vi "Register Events and Run.vi"(8 "error in (no error)":errorcluster, 11 "Panel in":refnum<class "Panel.lvclass">) -> (0 "error out":errorcluster, 2 "Panel Event Reg":refnum<event-registration>, 3 "Panel out":refnum<class "Panel.lvclass">)   [LabVIEW 2020, in "OOPanel.lvlib" / "Panel.lvclass"]
doc: "Simultaneously creates an event registration for the Panel events (Visibility, Close, etc) and marks the panel as running. Alternatively, Panel VIs can use the <b>Get Panel Events</b> property and then set the <b>Running</b> to true once the events are registered.\n\nFor more information on the <b>Running</b> property, see the VI documentation on <b>Set Running.vi</b>"
uses:
  Panel.lvclass
  Visibility State.ctl
  OOPanel.lvlib
  Visbility Event Data.ctl
  Panel Events.ctl
  Close Reason.ctl
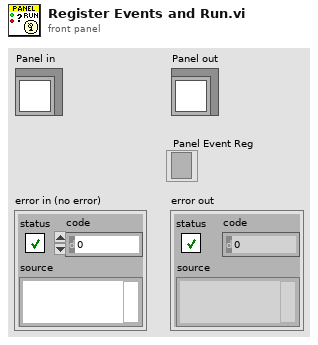
[diagram p1: front panel]
types:
  T1 = typedef "OOPanel.lvlib/Panel.lvclass/Panel Events.ctl" = cluster{"Visbility":refnum<user-event>, "Close":refnum<user-event>}
  T2 = typedef "OOPanel.lvlib/Panel.lvclass/Ref Data.ctl" = cluster{"Panel Ref":refnum<vi>, "SubPanel":refnum<vi>, "Close":bool, "Running":bool, "State":T3}
  T3 = typedef "OOPanel.lvlib/Visibility State.ctl" = enum16{"Idle", "Closed", "Hidden", "Visible", "Subpanel", "Hidden Subpanel"}
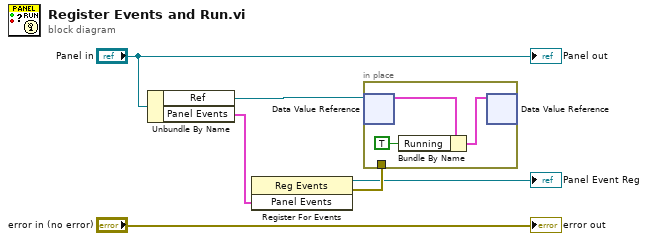
[diagram p0: block diagram]
diagram:
  n1 = Unbundle By Name("Panel in") -> ("Ref"=w5:refnum<data-value>, "Panel Events"=w1:T1)
  n2 = register-events(w1) -> (reference out=→"Panel Event Reg":refnum<event-registration>, error out=w3:errorcluster)  [unwired: 2 in]
  n3 = in-place {
    in-place-border: w3 -> [_]
    n4 = in-place-dvr #1(w5) -> (w9:T2)  [unwired: 1 out]
    n5 = Bundle By Name(cluster=w9, "Running"=TRUE) -> (w7:T2)
    n6 = in-place-dvr #1(w7) -> ()  [unwired: 2 out]
  }
  "error out" <- "error in (no error)"
  "Panel out" <- "Panel in"
